vi "api_GetString.vi"(7 "group":string, 8 "error in (no error)":errorcluster, 10 "param":string, 11 "ConfigClass_DVR":refnum<data-value>) -> (0 "error out":errorcluster, 2 "string_out":string, 3 "ConfigClass_DVR_out":refnum<data-value>)   [LabVIEW 2019, in "ConfigClass.lvlib" / "ConfigClass.lvclass"]
uses:
  ConfigClass.lvclass
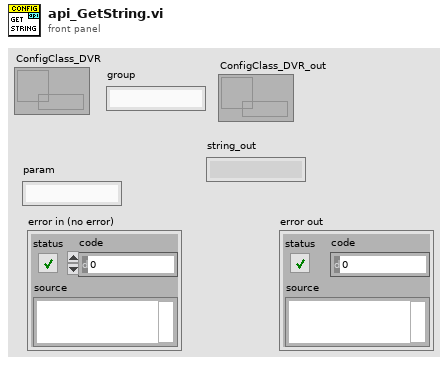
[diagram p1: front panel]
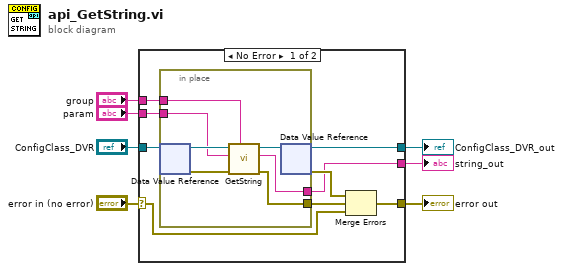
[diagram p0: block diagram]
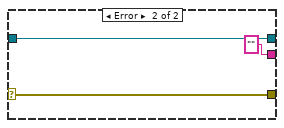
[diagram p2: hidden frame]
diagram:
  n1 = case shown="No Error" "error in (no error)" {
    selector: "error in (no error)" -> [w9 w26]
    tunnel: "ConfigClass_DVR" -> [w16 w25]
    tunnel: [w13 w26] -> w6
    tunnel: [w12 w25] -> w4
    tunnel: [w11 "" ("string_out")] -> w3
    tunnel: "group" -> [w10 _]
    tunnel: "param" -> [w8 _]
    frame No Error {
      n2 = in-place {
        in-place-border: [w20] -> w14
        in-place-border: [w19] -> w11
        in-place-border: w10 -> [w18]
        in-place-border: w8 -> [w17]
        n3 = in-place-dvr #1(w16) -> (w23:refnum<class "ConfigClass.lvclass">, w21:errorcluster)
        n4 = call-dynamic "GetString.vi"("group"=w18, "error in (no error)"=w21, "param"=w17, "ConfigClass_IN"=w23) -> ("error out"=w20:errorcluster, "string_out"=w19:string, "ConfigClass_OUT"=w22:refnum<class "ConfigClass.lvclass">)  [unwired: 5 in]
        n5 = in-place-dvr #1(w22) -> (w12:refnum<data-value>, w15:errorcluster)
      }
      n6 = Merge Errors(w15, w14, w9) -> (w13:errorcluster)
    }
    frame Error {
    }
  }
  "ConfigClass_DVR_out" <- w4
  "error out" <- w6
  "string_out" <- w3
